vi "read pressure.vi"() -> ()   [LabVIEW 2019]
uses:
  <vilib>/CANopenLib/CANOPEN.llb/CANopen Interface Create.vi
  <vilib>/CANopenLib/CANOPEN.llb/CANopen SDO Create.vi
  <vilib>/CANopenLib/CANOPEN.llb/CANopen Interface Close.vi
  <vilib>/CANopenLib/CANOPEN.llb/CANopen SDO Close.vi
  <vilib>/CANopenLib/CANOPEN.llb/CANopen SDO Read [U8].vi
panel:
  in  "interface name":u32(ring) items=["CANopen01", "CANopen02", "CANopen03", "CANopen04", "CANopen05", "CANopen06", "CANopen07", "CANopen08", "CANopen09", "CANopen10", "CANopen11", "CANopen12", "CANopen13", "CANopen14", "CANopen15", "CANopen16", "CANopen17", "CANopen18", "CANopen19", "CANopen20", "CANopen21", "CANopen22", "CANopen23", "CANopen24", "CANopen25", "CANopen26", "CANopen27", "CANopen28", "CANopen29", "CANopen30", "CANopen31", "CANopen32"]
  in  "Node ID":i8=1 min=1 max=10
  out "4-byte single":sgl
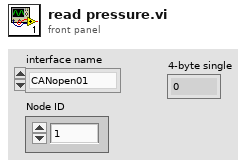
[diagram p1: front panel]
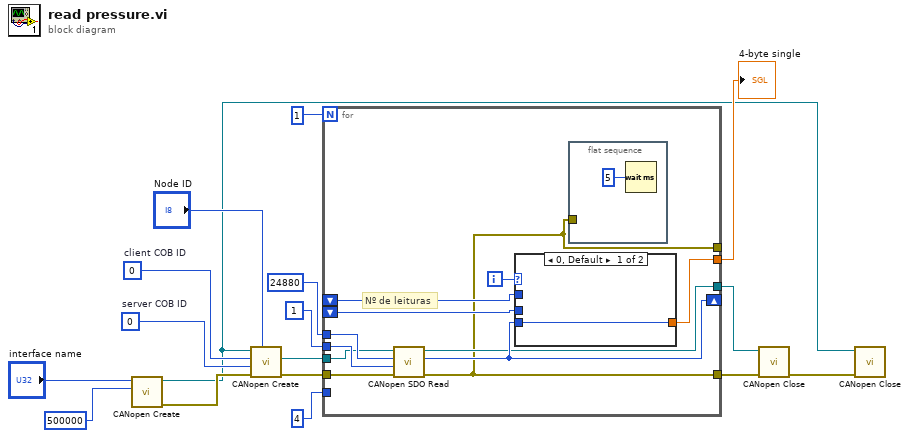
[diagram p0: block diagram]
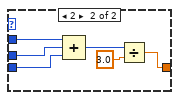
[diagram p2: hidden frame]
diagram:
  w7 = u32 0  # client COB ID
  w8 = u32 0  # server COB ID
  n1 = call-poly <vilib>:"CANopen Create.vi"("baud rate"=u32 500000 ("Baudrate"), "interface name"="interface name") -> ("error out"=w9:errorcluster, "interface object out"=w1:refnum<k20>)  [unwired: 8 in]
  n2 = call-poly <vilib>:"CANopen Create.vi"("node-ID"="Node ID", "error in (no error)"=w9, "server COB-ID (0)"=w8, "client COB-ID (0)"=w7, "interface object in"=w1) -> ("error out"=w6:errorcluster, "SDO object out"=w5:refnum<k20>)  [unwired: 4 in, 1 out]
  n3 = for {
    N: 1 -> [_]
    tunnel: w6 -> [w22]
    tunnel: u16 24880 ("object index") -> [w24]
    tunnel: u8 1 ("object sub-index (0)") -> [w23]
    tunnel: u32 4 ("data size") -> [_]
    tunnel: [w26] -> w17
    shift-right: [w20] -> _
    shift-left: _ -> [w28]
    shift-left: _ -> [w27]
    tunnel: [w18] -> _
    tunnel: w5 -> [w21]
    tunnel: [w18] -> w4
    tunnel: [w19] -> w2
    i -> [w25]
    # "Nº de leituras"
    n4 = call-poly <vilib>:"CANopen SDO Read.vi"("error in (no error)"=w22, "object sub-index (0)"=w23, "object index"=w24, "SDO object in"=w21) -> ("error out"=w18:errorcluster, "U8 data"=w20:u8, "SDO object out"=w19:refnum<k20>)  [unwired: 4 in, 1 out]
    n5 = case shown="0, Default" w25 {
      tunnel: w28 -> [_ w34]
      tunnel: w27 -> [_ w33]
      tunnel: w20 -> [w29 w32]
      tunnel: [w29 w30] -> w26
      frame 0, Default {
      }
      frame 2 {
        n6 = Compound Arithmetic op=ADD(w34, w33, w32) -> (w31:u8)
        n7 = Divide(x=w31, y=sgl 3.0) -> (x/y=w30:sgl)
      }
    }
    n8 = flat-sequence {
      tunnel: w18 -> [_]
      frame #0 {
        n9 = Wait (ms)(milliseconds to wait=u32 5) -> ()  [unwired: 1 out]
      }
    }
  }
  "4-byte single" <- w17
  n10 = call-poly <vilib>:"CANopen Close.vi"("error in (no error)"=w4, "SDO object in"=w2) -> ("error out"=w3:errorcluster)  [unwired: 9 in]
  n11 = call-poly <vilib>:"CANopen Close.vi"("error in (no error)"=w3, "interface object in"=w1) -> ()  [unwired: 9 in, 1 out]
